vi "Refresh Database Ports.vi"(8 "error in":errorcluster, 10 "Refresh Sysdef":T1[](array[typedef]), 11 "Database Ref":T5 format="%.0x") -> (0 "error out":errorcluster)   [LabVIEW 2020, in "Communication Bus Template System Explorer.lvlib" / "Implementation.lvlib"]
uses:
  Implementation.lvlib
  <vilib>/NI VeriStand/Custom Device API/Custom Device Item Ref.ctl
  Types/Refresh For Sysdef.ctl
  Types/Frame.ctl
  Types/Signal.ctl
  Types/ECU.ctl
  <vilib>/NI VeriStand/Custom Device Tools/Custom Device Utility Library/Search Direction.ctl
  <vilib>/NI VeriStand/Custom Device API/Custom Device Channel Type.ctl
  <vilib>/NI VeriStand/Custom Device API/Custom Device Channel.ctl
  Scripting/Constants.vi
  <vilib>/NI VeriStand/Custom Device Tools/Custom Device Utility Library/NI VeriStand - Search for Item by GUID.vi
  <vilib>/NI VeriStand/Custom Device Tools/Custom Device Utility Library/NI VeriStand - Search for All Items by GUID.vi
  Scripting/Communication Bus Template Scripting.lvlib
  <vilib>/NI VeriStand/Custom Device Tools/Custom Device Utility Library/Custom Device Utility Library.lvlib
  <vilib>/NI VeriStand/Custom Device API/Custom Device API.lvlib
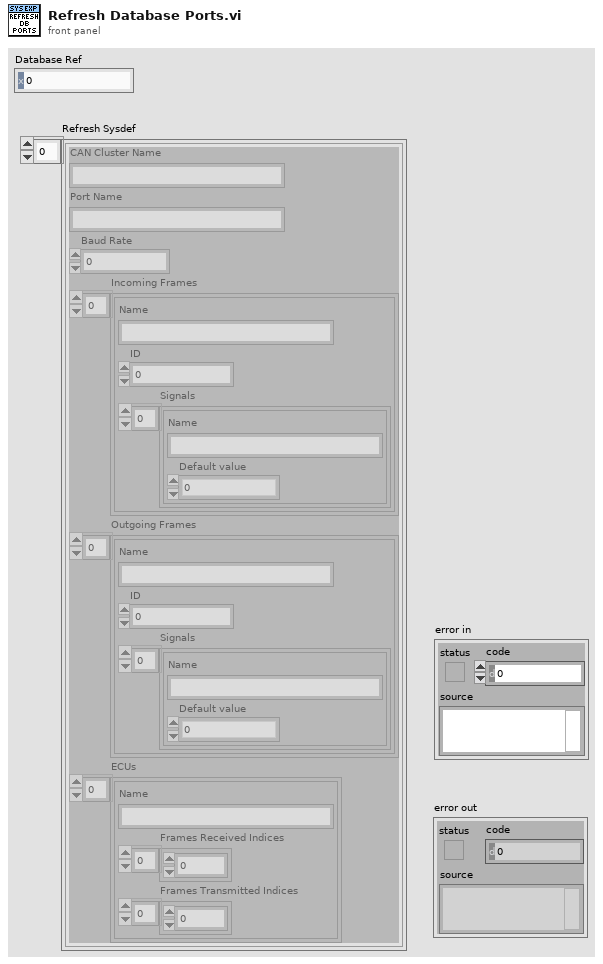
[diagram p1: front panel]
types:
  T1 = typedef "Communication Bus Template System Explorer.lvlib/Implementation.lvlib/Refresh For Sysdef.ctl" = cluster{"CAN Cluster Name":string, "Port Name":string, "Baud Rate":u64, "Incoming Frames":T2[], "Outgoing Frames":T2[], "ECUs":T4[]}
  T2 = typedef "Communication Bus Template System Explorer.lvlib/Implementation.lvlib/Frame.ctl" = cluster{"Name":string, "ID":u32, "Signals":T3[]}
  T3 = typedef "Communication Bus Template System Explorer.lvlib/Implementation.lvlib/Signal.ctl" = cluster{"Name":string, "Default value":dbl}
  T4 = typedef "Communication Bus Template System Explorer.lvlib/Implementation.lvlib/ECU.ctl" = cluster{"Name":string, "Frames Received Indices":u32[], "Frames Transmitted Indices":u32[]}
  T5 = typedef "Custom Device API.lvlib/Custom Device Item Ref.ctl" = u64
  T6 = typedef "Custom Device Utility Library.lvlib/Search Direction.ctl" = enum16{"Down", "Up"}
  T7 = typedef "Custom Device API.lvlib/Custom Device Channel Type.ctl" = enum16{"Input", "Output"}
  T8 = typedef "Custom Device API.lvlib/Custom Device Channel.ctl" = cluster{"Type":T7, "Units":string, "Default Value":dbl, "Faultable":bool, "Scalable":bool}
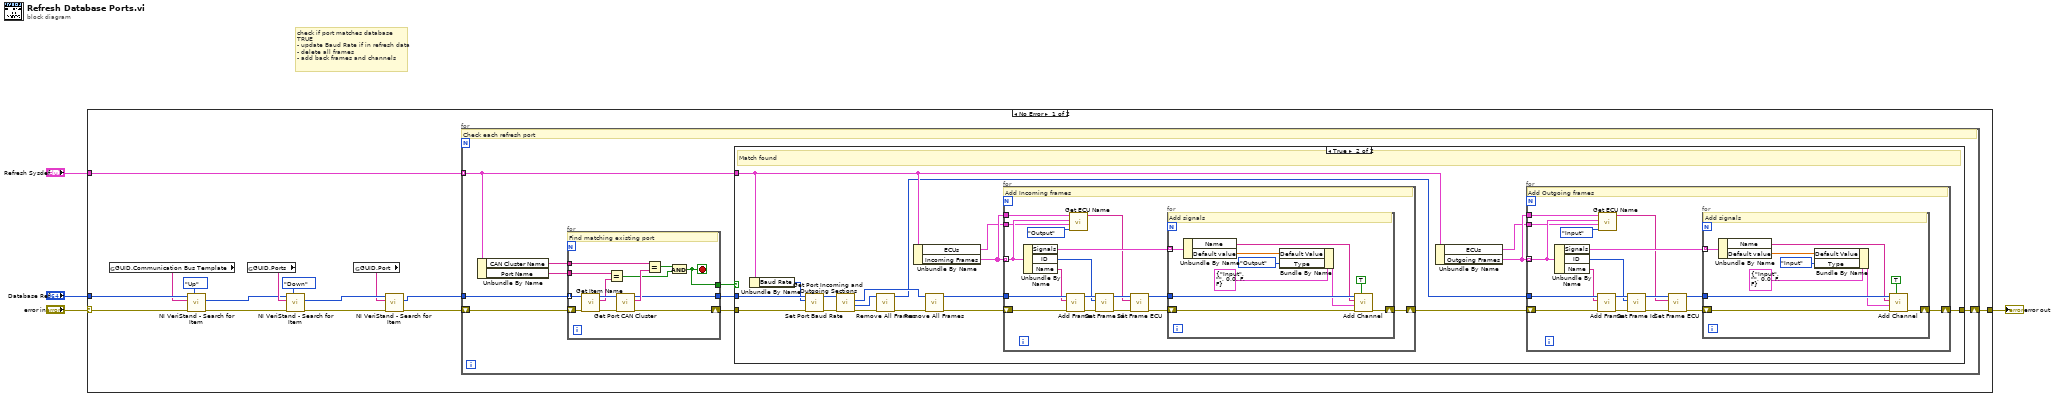
[diagram p0: block diagram]
diagram:
  # "check if port matches database\nTRUE\n- update Baud Rate if in refresh data\n- delete all frames\n- add back frames and channels"
  n1 = case shown="No Error" "error in" {
    selector: "error in" -> [w9 w116]
    tunnel: "Database Ref" -> [w19 _]
    tunnel: [w7 w116] -> w2
    tunnel: "Refresh Sysdef" -> [w5 _]
    frame No Error {
      n2 = global read "Constants.vi" "GUID.Communication Bus Template"() -> (w13:string)
      n3 = call-poly <vilib>:"NI VeriStand - Search for Item.vi"("Direction (Down)"=Search_Direction."Up", "error in"=w9, "Item GUID"=w13, "Section Ref in"=w19) -> ("error out"=w10:errorcluster, "Item Ref"=w11:T5)  [unwired: 4 in, 2 out]
      n4 = global read "Constants.vi" "GUID.Ports"() -> (w12:string)
      n5 = call-poly <vilib>:"NI VeriStand - Search for Item.vi"("Direction (Down)"=Search_Direction."Down", "error in"=w10, "Item GUID"=w12, "Section Ref in"=w11) -> ("error out"=w18:errorcluster, "Item Ref"=w17:T5)  [unwired: 4 in, 2 out]
      n6 = global read "Constants.vi" "GUID.Port"() -> (w16:string)
      n7 = call-poly <vilib>:"NI VeriStand - Search for Item.vi"("error in"=w18, "Item GUID"=w16, "Section Ref in"=w17) -> ("error out"=w8:errorcluster, "Item Refs"=w6:T5[])  [unwired: 5 in, 2 out]
      n8 = for {
        shift-right: [w20] -> w7
        shift-left: w8 -> [w28]
        tunnel: w5 -> [w21] mode=indexing
        tunnel: w6 -> [w27]
        # "Check each refresh port"
        n9 = Unbundle By Name(w21) -> ("CAN Cluster Name"=w26:string, "Port Name"=w25:string)
        n10 = for {
          tunnel: w27 -> [w112] mode=indexing
          tunnel: w26 -> [w109]
          tunnel: w25 -> [w111]
          tunnel: [w105] -> w23
          shift-right: [w104] -> w24
          shift-left: w28 -> [w113]
          tunnel: [w103] -> w22
          stop <- w103 stop-if-true
          # "Find matching existing port"
          n11 = call "Get Item Name.vi"("error in"=w113, "Item Ref"=w112) -> ("error out"=w114:errorcluster, "Name"=w110:string, "Item Ref out"=w115:T5)  [unwired: 7 in]
          n12 = Equal?(x=w111, y=w110) -> (x = y?=w106:bool)
          n13 = call "Get Port CAN Cluster.vi"("error in"=w114, "Port Ref"=w115) -> ("error out"=w104:errorcluster, "CAN Cluster"=w108:string, "Port Ref out"=w105:T5)  [unwired: 7 in]
          n14 = Equal?(x=w109, y=w108) -> (x = y?=w107:bool)
          n15 = And(x=w107, y=w106) -> (x .and. y?=w103:bool)
        }
        n16 = case shown="True" w22 {
          tunnel: w24 -> [w29 w42]
          tunnel: w23 -> [_ w44]
          tunnel: w21 -> [_ w39]
          tunnel: [w29 w34] -> w20
          frame False {
            # "We should never hit this case"
          }
          frame True {
            # "Match found"
            n17 = Unbundle By Name(w39) -> ("Baud Rate"=w41:u64)
            n18 = call "Set Port Baud Rate.vi"("error in"=w42, "Baud Rate"=w41, "Port Ref"=w44) -> ("error out"=w43:errorcluster, "Port Ref out"=w45:T5)  [unwired: 7 in]
            n19 = call "Get Port Incoming and Outgoing Sections.vi"("error in"=w43, "Port Ref"=w45) -> ("error out"=w48:errorcluster, "Outgoing"=w37:T5, "Incoming"=w46:T5)  [unwired: 6 in, 1 out]
            n20 = call "Remove All Frames.vi"("error in"=w48, "Incoming/Outgoing Ref"=w37) -> ("error out"=w47:errorcluster, "Incoming/Outgoing Ref out"=w36:T5)  [unwired: 8 in]
            n21 = Unbundle By Name(w39) -> ("ECUs"=w32:T4[], "Incoming Frames"=w33:T2[])
            n22 = call "Remove All Frames.vi"("error in"=w47, "Incoming/Outgoing Ref"=w46) -> ("error out"=w40:errorcluster, "Incoming/Outgoing Ref out"=w38:T5)  [unwired: 8 in]
            n23 = for {
              tunnel: w33 -> [w79] mode=indexing
              shift-right: [w85] -> w35
              shift-left: w40 -> [w92]
              tunnel: w38 -> [w91]
              tunnel: w33 -> [w80]
              tunnel: w32 -> [w78]
              # "Add Incoming frames"
              n24 = Unbundle By Name(w79) -> ("Signals"=w86:T3[], "ID"=w87:u32, "Name"=w90:string)
              n25 = call "Add Frame.vi"("error in"=w92, "Name"=w90, "Incoming/Outgoing Ref"=w91) -> ("error out"=w89:errorcluster, "Frame Ref out"=w88:T5)  [unwired: 6 in, 1 out]
              n26 = call "Get ECU Name.vi"("Type (Input)"=Custom_Device_Channel_Type."Output", "ECUs"=w78, "Frame"=w79, "Frames"=w80) -> ("ECU Name"=w77:string)  [unwired: 7 in]
              n27 = call "Set Frame Id.vi"("error in"=w89, "ID"=w87, "Frame Ref"=w88) -> ("error out"=w84:errorcluster, "Frame Ref out"=w83:T5)  [unwired: 7 in]
              n28 = call "Set Frame ECU.vi"("error in"=w84, "ECU Name"=w77, "Frame Ref"=w83) -> ("error out"=w81:errorcluster, "Frame Ref out"=w82:T5)  [unwired: 7 in]
              n29 = for {
                shift-right: [w101] -> w85
                shift-left: w81 -> [w102]
                tunnel: w82 -> [w100]
                tunnel: w86 -> [w99] mode=indexing
                # "Add signals"
                n30 = Unbundle By Name(w99) -> ("Name"=w98:string, "Default value"=w95:dbl)
                n31 = Bundle By Name(cluster=T8 {"Type"=enum."Input", "Units"="", "Default Value"=0.0, "Faultable"=FALSE, "Scalable"=FALSE} ("Channel"), "Default Value"=w95, "Type"=Custom_Device_Channel_Type."Output") -> (w94:T8)
                n32 = call "Add Channel.vi"("Highlight? (F)"=TRUE, "error in"=w102, "Channel"=w94, "Name"=w98, "Frame Ref"=w100) -> ("error out"=w101:errorcluster)  [unwired: 5 in, 1 out]
              }
            }
            n33 = Unbundle By Name(w39) -> ("ECUs"=w30:T4[], "Outgoing Frames"=w31:T2[])
            n34 = for {
              tunnel: w31 -> [w56] mode=indexing
              shift-right: [w58] -> w34
              shift-left: w35 -> [w65]
              tunnel: w36 -> [w64]
              tunnel: w31 -> [w57]
              tunnel: w30 -> [w55]
              # "Add Outgoing frames"
              n35 = Unbundle By Name(w56) -> ("Signals"=w59:T3[], "ID"=w60:u32, "Name"=w63:string)
              n36 = call "Add Frame.vi"("error in"=w65, "Name"=w63, "Incoming/Outgoing Ref"=w64) -> ("error out"=w62:errorcluster, "Frame Ref out"=w61:T5)  [unwired: 6 in, 1 out]
              n37 = call "Get ECU Name.vi"("Type (Input)"=Custom_Device_Channel_Type."Input", "ECUs"=w55, "Frame"=w56, "Frames"=w57) -> ("ECU Name"=w49:string)  [unwired: 7 in]
              n38 = call "Set Frame Id.vi"("error in"=w62, "ID"=w60, "Frame Ref"=w61) -> ("error out"=w51:errorcluster, "Frame Ref out"=w52:T5)  [unwired: 7 in]
              n39 = call "Set Frame ECU.vi"("error in"=w51, "ECU Name"=w49, "Frame Ref"=w52) -> ("error out"=w50:errorcluster, "Frame Ref out"=w53:T5)  [unwired: 7 in]
              n40 = for {
                shift-right: [w74] -> w58
                shift-left: w50 -> [w75]
                tunnel: w53 -> [w73]
                tunnel: w59 -> [w72] mode=indexing
                # "Add signals"
                n41 = Unbundle By Name(w72) -> ("Name"=w71:string, "Default value"=w68:dbl)
                n42 = Bundle By Name(cluster=T8 {"Type"=enum."Input", "Units"="", "Default Value"=0.0, "Faultable"=FALSE, "Scalable"=FALSE} ("Channel"), "Default Value"=w68, "Type"=Custom_Device_Channel_Type."Input") -> (w67:T8)
                n43 = call "Add Channel.vi"("Highlight? (F)"=TRUE, "error in"=w75, "Channel"=w67, "Name"=w71, "Frame Ref"=w73) -> ("error out"=w74:errorcluster)  [unwired: 5 in, 1 out]
              }
            }
          }
        }
      }
    }
    frame Error {
    }
  }
  "error out" <- w2
